vi "CheckIdPasswd(SubVI).vi"(1 "PIN":string, 2 "User Name":string) -> (0 "output":string)   [LabVIEW 2020]
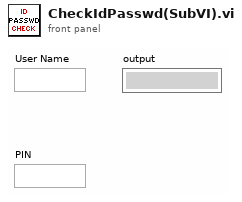
[diagram p1: front panel]
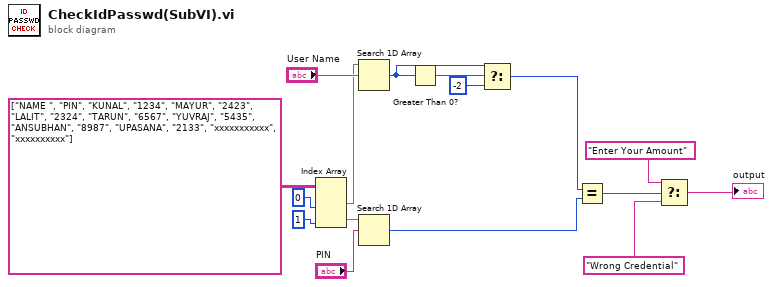
[diagram p0: block diagram]
diagram:
  n1 = Index Array(array=string[][] [["NAME ", "PIN"], ["KUNAL", "1234"], ["MAYUR", "2423"], ["LALIT", "2324"], ["TARUN", "6567"], ["YUVRAJ", "5435"], ["ANSUBHAN", "8987"], ["UPASANA", "2133"], ["xxxxxxxxxxx", "xxxxxxxxxx"]], index (col) #1=0 ("disabled index (col)"), index (col) #2=1 ("index (col)")) -> (element #1=w4:string[], element #2=w6:string[])  [unwired: 2 in]
  n2 = Search 1D Array(1D array=w4, element="User Name") -> (index of element=w9:i32)  [unwired: 1 in]
  n3 = Search 1D Array(1D array=w6, element="PIN") -> (index of element=w12:i32)  [unwired: 1 in]
  n4 = Greater Than 0?(x=w9) -> (x > 0?=w8:bool)
  n5 = Select(t=w9, s=w8, f=-2) -> (s? t:f=w11:i32)
  n6 = Equal?(x=w11, y=w12) -> (x = y?=w13:bool)
  n7 = Select(t="Enter Your Amount", s=w13, f="Wrong Credential") -> (s? t:f=→"output":string)
